vi "Launch One-Button Dialog Box.vi"(4 "Auto-stop? (T)":bool=TRUE, 5 "Return Priority (Normal)":T1=enum."Normal", 6 "Modal? (T)":bool=TRUE, 7 "Return Message (Optional)":refnum<class "Message.lvclass">, 8 "error in (no error)":errorcluster, 9 "Button Text (OK)":string="OK", 10 "Message Text":string, 11 "Dialog Launcher":refnum<class "IViewable.lvclass">) -> (0 "error out":errorcluster, 3 "Dialog Launcher Out":refnum<class "IViewable.lvclass">)   [LabVIEW 2020, in "OneButtonDialogBox.lvlib" / "OneButtonDialogBox.lvclass"]
doc: "启动单按钮对话框"
uses:
  OneButtonDialogBox.lvclass
  modules/mva-viewable/Source/IViewable/IViewable/IViewable.lvclass
  C:/Program Files/National Instruments/LabVIEW 2020/vi.lib/ActorFramework/Actor/Actor.lvclass
  <vilib>/ActorFramework/Message/Message.lvclass
  <vilib>/ActorFramework/Message Enqueuer/Message Priority.ctl
  <vilib>/ActorFramework/Actor/Actor.lvclass/Actor.ctl
  <vilib>/ActorFramework/Message Enqueuer/Message Enqueuer.lvclass/Message Enqueuer.ctl
  IDialogBox/IDialogBox Messages/Dialog Return Msg/Dialog Return Msg.lvclass/Dialog Return Msg.ctl
  OneButtonDialogBox.lvclass/OneButtonDialogBox.ctl
  <vilib>/ActorFramework/Message Enqueuer/Init from Existing Queue.vi
  <vilib>/ActorFramework/Message Enqueuer/Message Enqueuer.lvclass
  IDialogBox/IDialogBox Messages/Dialog Return Msg/Dialog Return Msg.lvclass
  <vilib>/ActorFramework/Actor/Actor.lvclass
  IDialogBox/IDialogBox/IDialogBox.lvclass
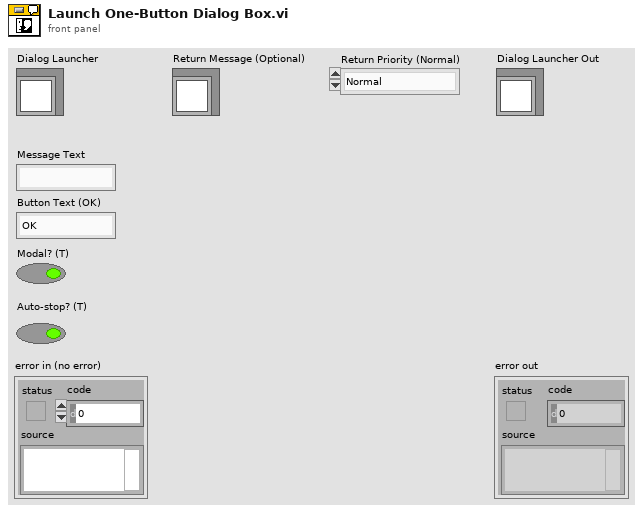
[diagram p1: front panel]
types:
  T1 = typedef "Actor Framework.lvlib/Message Enqueuer.lvclass/Message Priority.ctl" = enum16{"Low", "Normal", "High"}
  T2 = enum32{"Invalid", "Default", "Floating", "Floating/Auto-Hide", "Modal"}
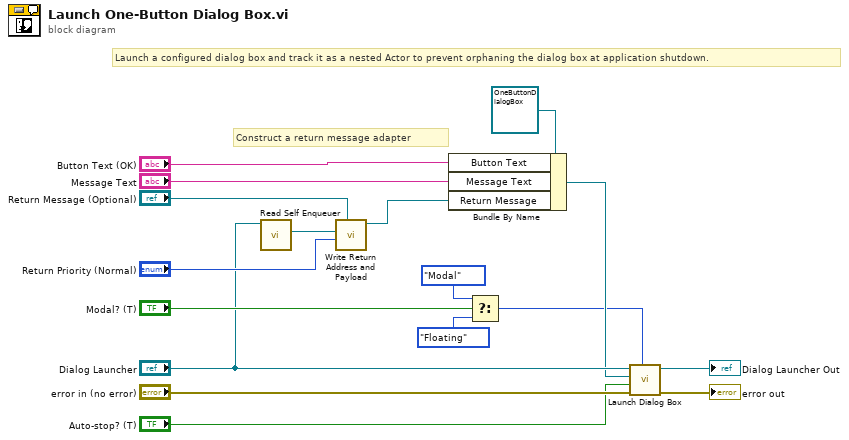
[diagram p0: block diagram]
diagram:
  # "Construct a return message adapter"
  # "Launch a configured dialog box and track it as a nested Actor to prevent orphaning the dialog box at application shutdown."
  n1 = call <vilib>:"Read Self Enqueuer.vi"("Actor"="Dialog Launcher") -> ("Self Enqueuer"=w5:refnum<class "Message Enqueuer.lvclass">)  [unwired: 10 in]
  n2 = call "Write Return Address and Payload.vi"("Reply Message"="Return Message (Optional)", "Return Priority (Normal)"="Return Priority (Normal)", "Return Address"=w5) -> ("Dialog Return Msg out"=w6:refnum<class "Dialog Return Msg.lvclass">)  [unwired: 8 in]
  n3 = Bundle By Name(cluster=refnum<class "OneButtonDialogBox.lvclass"> refnum ("OneButtonDialogBox in"), "Button Text"="Button Text (OK)", "Message Text"="Message Text", "Return Message"=w6) -> (w2:refnum<class "OneButtonDialogBox.lvclass">)
  n4 = Select(t=T2."Modal" ("FP Window:Behavior"), s="Modal? (T)", f=T2."Floating" ("FP Window:Behavior")) -> (s? t:f=w1:T2)
  n5 = call "Launch Dialog Box.vi"("FP Window:Behavior (Floating)"=w1, "error in (no error)"="error in (no error)", "Auto-stop? (T)"="Auto-stop? (T)", "DialogBox"=w2, "DialogBox Launcher"="Dialog Launcher") -> ("error out"=→"error out":errorcluster, "DialogBox Launcher"=→"Dialog Launcher Out":refnum<class "IViewable.lvclass">)  [unwired: 4 in, 1 out]
